vi "Read perform dynamic writes.vi"(8 "error in":errorcluster, 11 "DecideProjectFeatures in":refnum<class "TagBusProcessingPluginFeatureDecider.lvclass">) -> (0 "error out":errorcluster, 2 "perform dynamic writes":bool, 3 "DecideProjectFeatures out":refnum<class "TagBusProcessingPluginFeatureDecider.lvclass">)   [LabVIEW 2013, in "TagBusProcessingPluginFeatureDecider.lvclass"]
uses:
  TagBusProcessingPluginFeatureDecider.lvclass
  TagBusProcessingPluginFeatureDecider.lvclass/TagBusProcessingPluginFeatureDecider.ctl
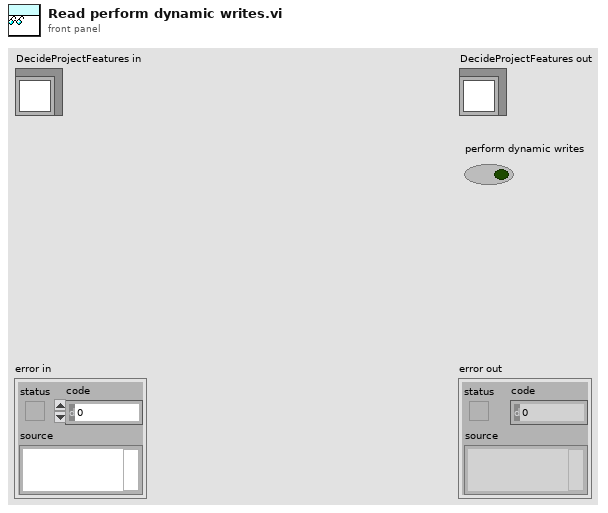
[diagram p1: front panel]
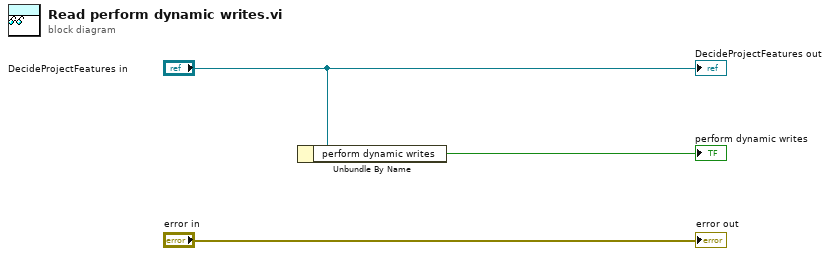
[diagram p0: block diagram]
diagram:
  n1 = Unbundle By Name("DecideProjectFeatures in") -> ("perform dynamic writes"=→"perform dynamic writes":bool)
  "error out" <- "error in"
  "DecideProjectFeatures out" <- "DecideProjectFeatures in"
